vi "Camera Configuration.vi"(8 "error in (no error)":errorcluster, 11 "CCDCamera in":refnum<class "CCDCamera.lvclass">) -> (0 "error out":errorcluster, 3 "CCDCamera out":refnum<class "CCDCamera.lvclass">)   [LabVIEW 2018, in "CCDCamera.lvclass"]
doc: "Este VI faz a leitura de todos os parâmetros de configuração salvos na classe e os escreve na câmera."
uses:
  CCDCamera.lvclass
  CCDCamera.lvclass/CCDCamera.ctl
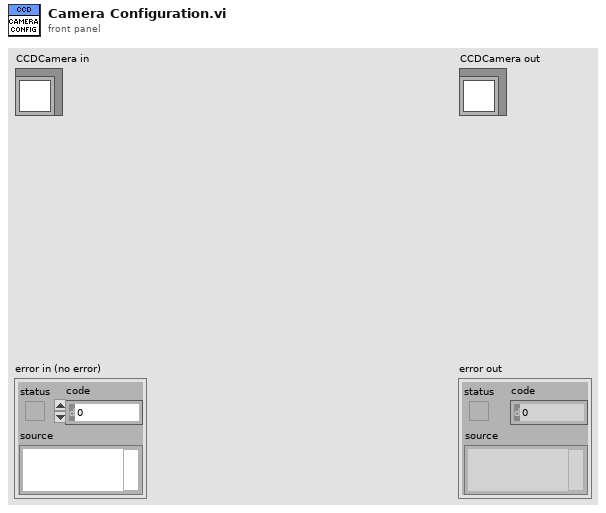
[diagram p1: front panel]
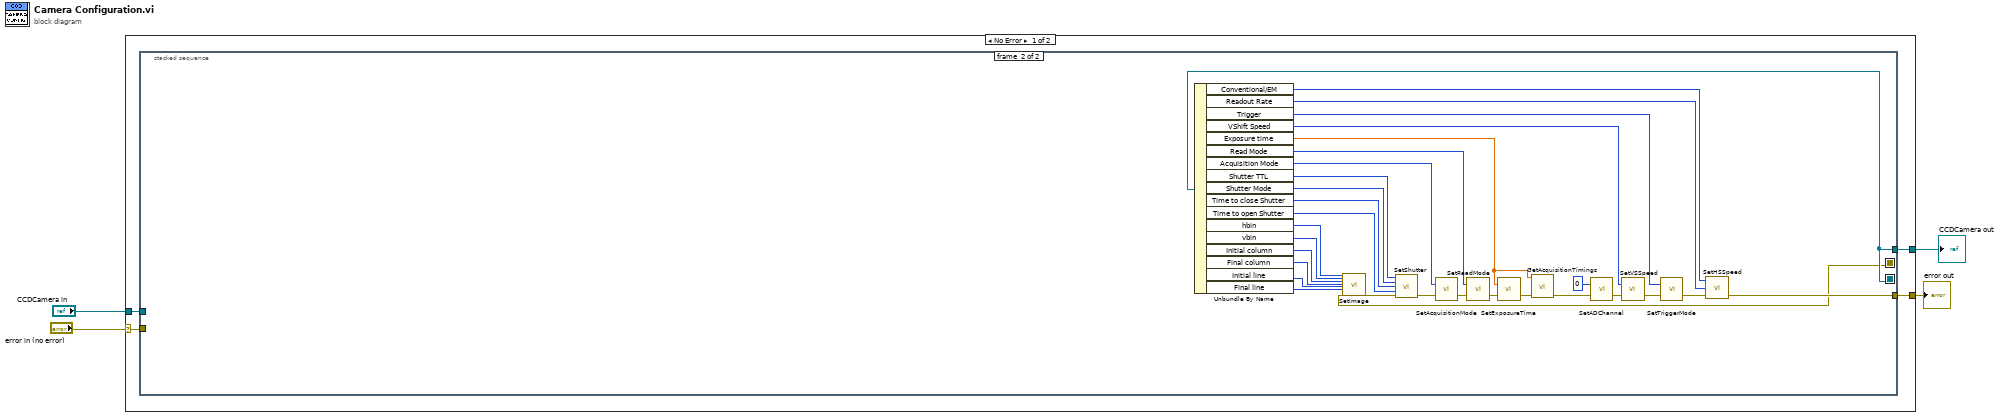
[diagram p0: block diagram]
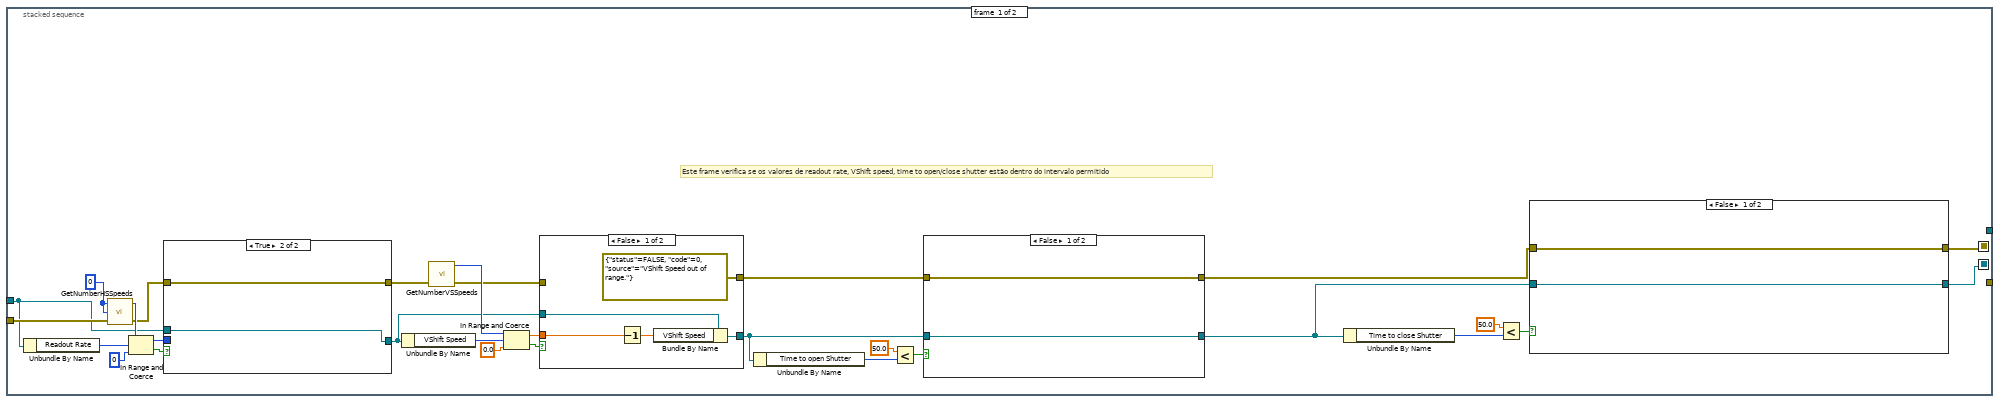
[diagram p2: hidden frame]
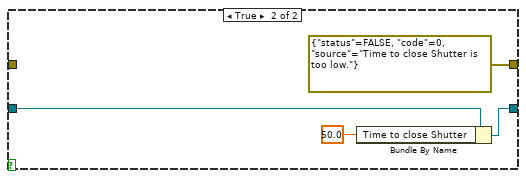
[diagram p3: hidden frame]
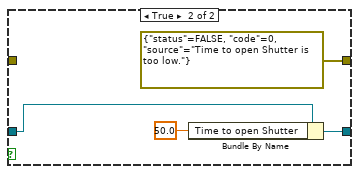
[diagram p4: hidden frame]
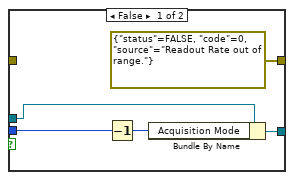
[diagram p6: hidden frame]
diagram:
  n1 = case shown="No Error" "error in (no error)" {
    selector: "error in (no error)" -> [w7 w95]
    tunnel: [w6 w95] -> w3
    tunnel: [w5 w94] -> w1
    tunnel: "CCDCamera in" -> [w8 w94]
    frame No Error {
      n2 = stacked-sequence {
        seq-local: [w11 _] -> [_ w67]
        seq-local: [w12 _] -> [_ w68]
        tunnel: w8 -> [w9 _]
        tunnel: w7 -> [w10 _]
        tunnel: [_ w69] -> w6
        tunnel: [_ w68] -> w5
        frame #0 {
          w37 = 0 ("channel")
          # "Este frame verifica se os valores de readout rate, VShift speed, time to open/close shutter estão dentro do intervalo permitido"
          n3 = Unbundle By Name(w9) -> ("Readout Rate"=w34:u16)
          n4 = call <userlib>:"GetNumberHSSpeeds.vi"("error in (no error)"=w10, "type"=w37, "channel"=w37) -> ("error out"=w31:errorcluster, "number"=w35:i32)  [unwired: 1 out]
          n5 = In Range and Coerce(upper limit=w35, x=w34, lower limit=0 ("channel")) -> (coerced(x)=w32:i32, In Range?=w33:bool)
          n6 = case shown="True" w33 {
            tunnel: w32 -> [w61 _]
            tunnel: w9 -> [w60 w63]
            tunnel: w31 -> [_ w62]
            tunnel: [errorcluster {"status"=FALSE, "code"=0, "source"="Readout Rate out of range."} ("error out") w62] -> w27
            tunnel: [w57 w63] -> w23
            frame False {
              n7 = Decrement(x=w61) -> (x-1=w59:i32)
              n8 = Bundle By Name(cluster=w60, "Acquisition Mode"=w59) -> (w57:refnum<class "CCDCamera.lvclass">)
            }
            frame True {
            }
          }
          n9 = Unbundle By Name(w23) -> ("VShift Speed"=w29:u16)
          n10 = call <userlib>:"GetNumberVSSpeeds.vi"("error in (no error)"=w27) -> ("error out"=w24:errorcluster, "number"=w28:i32)  [unwired: 2 in, 1 out]
          n11 = In Range and Coerce(upper limit=w28, x=w29, lower limit=0.0) -> (coerced(x)=w25:dbl, In Range?=w26:bool)
          n12 = case shown="False" w26 {
            tunnel: w25 -> [w54 _]
            tunnel: w23 -> [w53 w56]
            tunnel: w24 -> [_ w55]
            tunnel: [errorcluster {"status"=FALSE, "code"=0, "source"="VShift Speed out of range."} ("error out") w55] -> w18
            tunnel: [w50 w56] -> w20
            frame False {
              n13 = Decrement(x=w54) -> (x-1=w52:dbl)
              n14 = Bundle By Name(cluster=w53, "VShift Speed"=w52) -> (w50:refnum<class "CCDCamera.lvclass">)
            }
            frame True {
            }
          }
          n15 = Unbundle By Name(w20) -> ("Time to open Shutter"=w21:u16)
          n16 = Less?(x=50.0, y=w21) -> (x < y?=w19:bool)
          n17 = case shown="False" w19 {
            tunnel: w20 -> [w45 w49]
            tunnel: [w44 errorcluster {"status"=FALSE, "code"=0, "source"="Time to open Shutter is too low."} ("error out")] -> w13
            tunnel: [w45 w46] -> w14
            tunnel: w18 -> [w44 _]
            frame False {
            }
            frame True {
              n18 = Bundle By Name(cluster=w49, "Time to open Shutter"=50.0) -> (w46:refnum<class "CCDCamera.lvclass">)
            }
          }
          n19 = Unbundle By Name(w14) -> ("Time to close Shutter"=w16:u16)
          n20 = Less?(x=50.0, y=w16) -> (x < y?=w17:bool)
          n21 = case shown="False" w17 {
            tunnel: w14 -> [w39 w43]
            tunnel: [w38 errorcluster {"status"=FALSE, "code"=0, "source"="Time to close Shutter is too low."} ("error out")] -> w11
            tunnel: [w39 w40] -> w12
            tunnel: w13 -> [w38 _]
            frame False {
            }
            frame True {
              n22 = Bundle By Name(cluster=w43, "Time to close Shutter"=50.0 ("Time to open Shutter")) -> (w40:refnum<class "CCDCamera.lvclass">)
            }
          }
        }
        frame #1 {
          n23 = Unbundle By Name(w68) -> ("Conventional/EM"=w70:u16, "Readout Rate"=w71:u16, "Trigger"=w72:u16, "VShift Speed"=w73:u16, "Exposure time"=w64:dbl, "Read Mode"=w74:u16, "Acquisition Mode"=w75:u16, "Shutter TTL"=w78:u16, "Shutter Mode"=w79:u16, "Time to close Shutter"=w80:u16, "Time to open Shutter"=w81:u16, "hbin"=w82:u16, "vbin"=w83:u16, "Initial column"=w84:u16, "Final column"=w85:u32, "Initial line"=w86:u16, "Final line"=w87:u32)
          n24 = call <userlib>:"SetImage.vi"("hbin"=w82, "vbin"=w83, "hstart"=w84, "hend"=w85, "vstart"=w86, "vend"=w87, "error in (no error)"=w67) -> ("error out"=w77:errorcluster)  [unwired: 19 in, 1 out]
          n25 = call <userlib>:"SetShutter.vi"("type"=w78, "mode"=w79, "closingtime"=w80, "openingtime"=w81, "error in (no error)"=w77) -> ("error out"=w76:errorcluster)  [unwired: 9 in, 1 out]
          n26 = call <userlib>:"SetAcquisitionMode.vi"("error in (no error)"=w76, "mode"=w75) -> ("error out"=w93:errorcluster)  [unwired: 1 out]
          n27 = call <userlib>:"SetReadMode.vi"("error in (no error)"=w93, "mode"=w74) -> ("error out"=w92:errorcluster)  [unwired: 1 out]
          n28 = call <userlib>:"SetExposureTime.vi"("error in (no error)"=w92, "time"=w64) -> ("error out"=w66:errorcluster)  [unwired: 1 out]
          n29 = call <userlib>:"GetAcquisitionTimings.vi"("exposure input"=w64, "error in (no error)"=w66) -> ("error out"=w65:errorcluster)  [unwired: 9 in, 4 out]
          n30 = call <userlib>:"SetADChannel.vi"("error in (no error)"=w65, "channel"=0) -> ("error out"=w91:errorcluster)  [unwired: 1 out]
          n31 = call <userlib>:"SetVSSpeed.vi"("error in (no error)"=w91, "index"=w73) -> ("error out"=w90:errorcluster)  [unwired: 1 out]
          n32 = call <userlib>:"SetTriggerMode.vi"("error in (no error)"=w90, "mode"=w72) -> ("error out"=w89:errorcluster)  [unwired: 1 out]
          n33 = call <userlib>:"SetHSSpeed.vi"("error in (no error)"=w89, "index"=w71, "type"=w70) -> ("error out"=w69:errorcluster)  [unwired: 1 in, 1 out]
        }
      }
    }
    frame Error {
    }
  }
  "error out" <- w3
  "CCDCamera out" <- w1
